vi "Teleop.vi"(10 "Match Info":T1={"Autonomous Elapsed Seconds"=0.0, "TeleOp Elapsed Seconds"=0.0, "Disabled Elapsed Seconds"=0.0, "Visited Autonomous"=FALSE, "Visited TeleOp"=FALSE, "Visited Disabled"=FALSE, "Autonomous Settings"={"Autonomous Style"=enum."Independent", "VI Refnum"=refnum}}, 11 "Call Context":T2) -> ()   [LabVIEW 2015]
doc: "This VI is called for each TeleOp packet received from the DS where the robot is not disabled. It is often used to read from the joysticks and update I/O or to update setpoints for timed control loops. It should complete and return within 20 milliseconds or it may miss DS packets."
uses:
  <vilib>/Rock Robotics/WPI/DriverStation/WPI_DriverStationDerivedRobotMode.ctl
  <vilib>/Rock Robotics/WPI/DriverStation/WPI_DriverStationMatch Info.ctl
  <vilib>/Rock Robotics/WPI/Relay/WPI_RelayValue.ctl
  <vilib>/Rock Robotics/WPI/Utilities/WPI_GetSetVariantRefNum.vi
  <vilib>/Rock Robotics/Network Tables/NT Write Number.vi
  <vilib>/Rock Robotics/Network Tables/NT Write Boolean Array.vi
  <vilib>/Rock Robotics/Network Tables/NT Write Numeric Array.vi
  <vilib>/Rock Robotics/Network Tables/NT Read Number.vi
  Robot Global Data.vi
  <vilib>/Rock Robotics/Network Tables/NT Write Boolean.vi
  <vilib>/Rock Robotics/WPI/RobotDrive/WPI_RobotDriveArcadeDrive_Standard(NoSaturation).vi
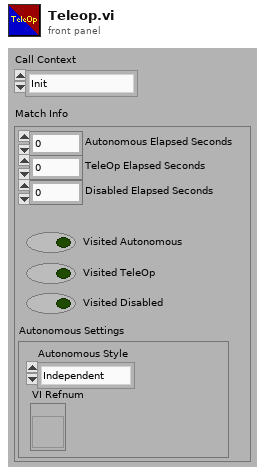
[diagram p1: front panel]
types:
  T1 = typedef "WPI_DriverStationMatch Info.ctl" = cluster{"Autonomous Elapsed Seconds":dbl, "TeleOp Elapsed Seconds":dbl, "Disabled Elapsed Seconds":dbl, "Visited Autonomous":bool, "Visited TeleOp":bool, "Visited Disabled":bool, "Autonomous Settings":cluster{"Autonomous Style":enum16{"Iterative", "Independent"}, "VI Refnum":refnum<vi>}}
  T2 = typedef "WPI_DriverStationDerivedRobotMode.ctl" = enum16{"Init", "Execute", "Stop"}
  T3 = typedef "WPI_RelayValue.ctl" = enum16{"Off", "On", "Forward", "Reverse"}
  T4 = typedef "WPI_JoystickDevRef.ctl" = cluster{"Device":T5}
  T5 = typedef "WPI_JoystickDeviceEnum.ctl" = enum16{"USB 0", "USB 1", "USB 2", "USB 3", "USB 4", "USB 5"}
  T6 = typedef "WPI_ServoDeviceRef.ctl" = cluster{"DeviceStatus":errorcluster, "PWM Channel":T7, "DeadBand":T8}
  T7 = typedef "FPGA_DIOPWMChannel.ctl" = enum8{"PWM 0", "PWM 1", "PWM 2", "PWM 3", "PWM 4", "PWM 5", "PWM 6", "PWM 7", "PWM 8", "PWM 9", "PWM MXP 0", "PWM MXP 1", "PWM MXP 2", "PWM MXP 3", "PWM MXP 4", "PWM MXP 5", "PWM MXP 6", "PWM MXP 7", "PWM MXP 8", "PWM MXP 9", "Invalid"}
  T8 = typedef "WPI_PWMDeadband.ctl" = cluster{"Name":string, "maxPositivePwm":i32, "minPositivePwm":i32, "centerPwm":i32, "maxNegativePwm":i32, "minNegativePwm":i32, "angularRange":u16}
  T9 = typedef "WPI_RobotDriveDevRef.ctl" = cluster{"DevStatus":errorcluster, "Motors[]":T10[], "Square Inputs":bool, "Max Output":dbl}
  T10 = typedef "WPI_MotorControlDeviceRef.ctl" = cluster{"DeviceStatus":errorcluster, "Type":T11, "PWM":cluster{"PWM Channel":T7, "DeadBand":T8}, "CAN":cluster{"Device Number":u8, "Control Mode":T12, "Semaphore":T13, "Max Vout":dbl, "TalonSRX Control Mode":T14}, "Invert":bool}
  T11 = typedef "WPI_MotorControlType.ctl" = enum16{"PWM", "CAN", "CANTalonSRX"}
  T12 = typedef "WPI_CANJaguar_ControlMode.ctl" = enum8{"Percent VBus", "Current", "Speed", "Position", "Voltage"}
  T13 = typedef "Semaphore RefNum" = refnum<k1>
  T14 = typedef "WPI_CANTalonSRX_APIControlMode.ctl" = enum8{"Percent VBus", "Speed", "Position", "Slave", "Unchanged / Invalid", "Voltage Compensation", "Current", "Motion Profile"}
  T15 = typedef "WPI_RelayDevRef.ctl" = cluster{"DevStatus":errorcluster, "Relay Channel":T16, "Relay Direction":T17}
  T16 = typedef "FPGA_DIORelayChannel.ctl" = enum8{"Relay 0", "Relay 1", "Relay 2", "Relay 3", "Invalid"}
  T17 = typedef "WPI_RelayDirection.ctl" = enum16{"Both directions", "Forward only", "Reverse only"}
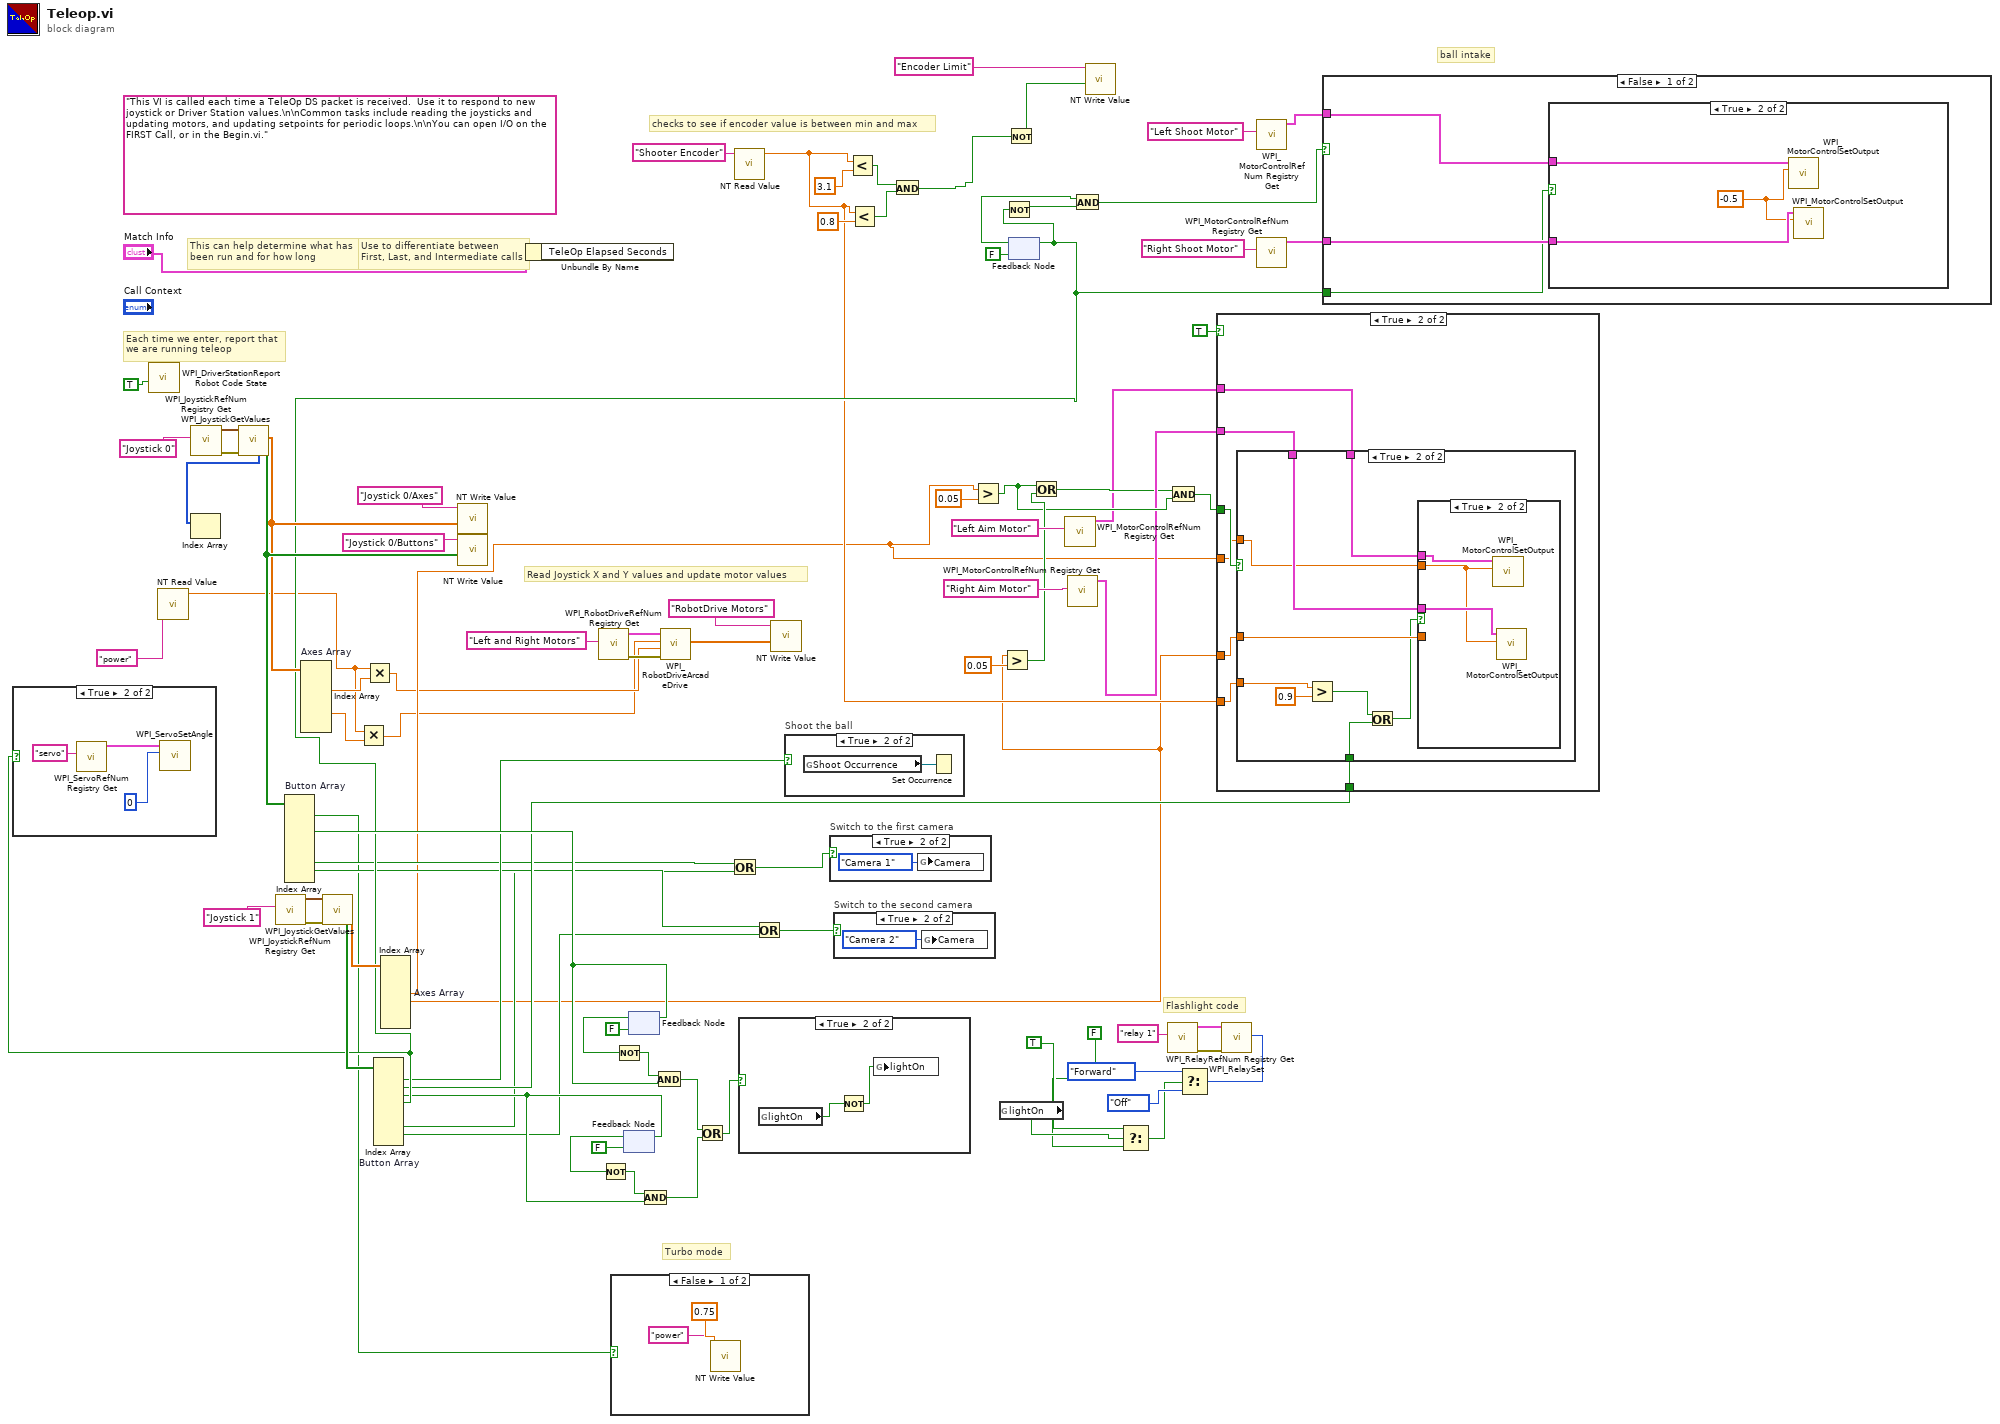
[diagram p0: block diagram]
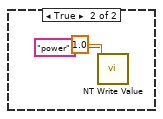
[diagram p2: hidden frame]
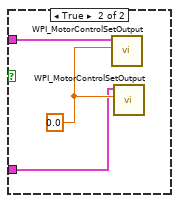
[diagram p5: hidden frame]
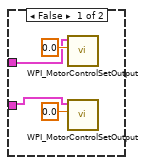
[diagram p7: hidden frame]
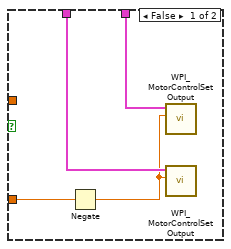
[diagram p8: hidden frame]
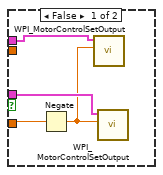
[diagram p9: hidden frame]
diagram:
  (unwired) "This VI is called each time a TeleOp DS packet is received.  Use it to respond to new joystick or Driver Station values.\n\nCommon tasks include reading the joysticks and updating motors, and updating setpoints for periodic loops.\n\nYou can open I/O on the FIRST Call, or in the Begin.vi."
  # "Turbo mode"
  # "ball intake"
  # "Flashlight code"
  # "checks to see if encoder value is between min and max"
  # "Each time we enter, report that\nwe are running teleop"
  # "Use to differentiate between\nFirst, Last, and Intermediate calls"
  # "This can help determine what has\nbeen run and for how long"
  # "Read Joystick X and Y values and update motor values"
  n1 = call <vilib>:"WPI_DriverStationReport Robot Code State.vi"("TeleOp"=TRUE ("Autonomous")) -> ()  [unwired: 10 in, 1 out]
  n2 = call-poly <vilib>:"NT Read Value.vi"("Name"="power") -> ("Numeric"=w3:dbl)  [unwired: 9 in, 1 out]
  n3 = call <vilib>:"WPI_JoystickRefNum Registry Get.vi"("refnum name"="Joystick 0") -> ("error out"=w76:errorcluster, "JoystickDevRef"=w82:T4)  [unwired: 1 in, 8 out]
  n4 = call <vilib>:"WPI_JoystickGetValues.vi"("error in (no error)"=w76, "JoystickDevRef"=w82) -> ("Buttons"=w77:bool[], "Axes"=w74:dbl[], "POVs"=w16:i16[])  [unwired: 5 in, 2 out]
  n5 = Index Array(array=w16) -> ()  [unwired: 1 in, 1 out]
  n6 = call <vilib>:"WPI_JoystickRefNum Registry Get.vi"("refnum name"="Joystick 1") -> ("error out"=w51:errorcluster, "JoystickDevRef"=w53:T4)  [unwired: 1 in, 8 out]
  n7 = Index Array "Button Array"(array=w77) -> (element #1=w9:bool, element #3=w55:bool, element #7=w11:bool, element #8=w14:bool)  [unwired: 9 in, 5 out]
  n8 = Index Array "Axes Array"(array=w74) -> (element #2=w5:dbl, element #5=w2:dbl)  [unwired: 7 in, 5 out]
  n9 = call <vilib>:"WPI_JoystickGetValues.vi"("error in (no error)"=w51, "JoystickDevRef"=w53) -> ("Buttons"=w52:bool[], "Axes"=w50:dbl[])  [unwired: 5 in, 3 out]
  n10 = Multiply(x=w3, y=w2) -> (x*y=w1:dbl)
  n11 = Multiply(x=w3, y=w5) -> (x*y=w4:dbl)
  n12 = Index Array "Button Array"(array=w52) -> (element #1=w26:bool, element #2=w17:bool, element #3=w22:bool, element #4=w27:bool, element #7=w12:bool, element #8=w15:bool)  [unwired: 9 in, 3 out]
  n13 = case shown="True" w27 {
    frame False {
    }
    frame True {
      n14 = call <vilib>:"WPI_ServoRefNum Registry Get.vi"("refnum name"="servo") -> ("ServoDeviceRef"=w89:T6)  [unwired: 9 in, 1 out]
      n15 = call <vilib>:"WPI_ServoSetAngle.vi"("Angle"=0, "ServoDeviceRef"=w89) -> ()  [unwired: 8 in, 2 out]
    }
  }
  n16 = Index Array "Axes Array"(array=w50) -> (element #3=w6:dbl, element #4=w7:dbl)  [unwired: 7 in, 5 out]
  n17 = call-poly <vilib>:"NT Write Value.vi"("Numeric Array"=w74, "Name"="Joystick 0/Axes") -> ()  [unwired: 9 in, 1 out]
  n18 = call-poly <vilib>:"NT Write Value.vi"("Boolean Array"=w77, "Name"="Joystick 0/Buttons") -> ()  [unwired: 9 in, 1 out]
  n19 = Unbundle By Name("Match Info") -> ()  [unwired: 1 out]
  n20 = call <vilib>:"WPI_RobotDriveRefNum Registry Get.vi"("refnum name"="Left and Right Motors") -> ("error out"=w75:errorcluster, "RobotDriveDevRef"=w84:T9)  [unwired: 1 in, 8 out]
  n21 = case shown="False" w9 {
    frame False {
      n22 = call-poly <vilib>:"NT Write Value.vi"("Numeric"=0.75, "Name"="power") -> ()  [unwired: 9 in, 1 out]
    }
    frame True {
      n23 = call-poly <vilib>:"NT Write Value.vi"("Numeric"=1.0, "Name"="power") -> ()  [unwired: 9 in, 1 out]
    }
  }
  n24 = feedback #1(FALSE) -> (w24:bool)
  n25 = Not(x=w24) -> (.not. x?=w23:bool)
  n26 = feedback-in #1(w22) -> ()
  n27 = feedback #2(FALSE) -> (w57:bool)
  n28 = Not(x=w57) -> (.not. x?=w56:bool)
  n29 = feedback-in #2(w55) -> ()
  n30 = And(x=w23, y=w22) -> (x .and. y?=w20:bool)
  n31 = And(x=w56, y=w55) -> (x .and. y?=w21:bool)
  n32 = call-poly <vilib>:"WPI_RobotDriveArcadeDrive.vi"("error in (no error)"=w75, "Y axis value"=w4, "X axis value"=w1, "RobotDriveDevRef"=w84) -> ("Motor Values"=w79:dbl[])  [unwired: 5 in, 2 out]
  n33 = Or(x=w21, y=w20) -> (x .or. y?=w19:bool)
  n34 = Or(x=w11, y=w12) -> (x .or. y?=w10:bool)
  n35 = call-poly <vilib>:"NT Read Value.vi"("Name"="Shooter Encoder" ("refnum name")) -> ("Numeric"=w18:dbl)  [unwired: 9 in, 1 out]
  n36 = case shown="True" w19 {
    frame False {
    }
    frame True {
      n37 = global read "Robot Global Data.vi" "lightOn"() -> (w96:bool)
      n38 = Not(x=w96) -> (.not. x?=w95:bool)
      n39 = global write "Robot Global Data.vi" "lightOn"(w95) -> ()
    }
  }
  n40 = Or(x=w14, y=w15) -> (x .or. y?=w13:bool)
  n41 = call-poly <vilib>:"NT Write Value.vi"("Numeric Array"=w79, "Name"="RobotDrive Motors") -> ()  [unwired: 9 in, 1 out]
  n42 = case "Shoot the ball" shown="True" w26 {
    frame False {
    }
    frame True {
      n43 = global read "Robot Global Data.vi" "Shoot Occurrence"() -> (w97:refnum<k4>)
      n44 = Set Occurrence(w97) -> ()
    }
  }
  n45 = case "Switch to the first camera" shown="True" w10 {
    frame False {
    }
    frame True {
      n46 = global write "Robot Global Data.vi" "Camera"(enum16{"Camera 1", "Camera 2"}."Camera 1" ("Camera")) -> ()
    }
  }
  n47 = case "Switch to the second camera" shown="True" w13 {
    frame False {
    }
    frame True {
      n48 = global write "Robot Global Data.vi" "Camera"(enum16{"Camera 1", "Camera 2"}."Camera 2" ("Camera")) -> ()
    }
  }
  n49 = Less?(x=w18, y=3.1) -> (x < y?=w41:bool)
  n50 = Less?(x=w18, y=0.8) -> (x < y?=w40:bool)
  n51 = And(x=w41, y=w40) -> (x .and. y?=w39:bool)
  n52 = Greater?(x=w6, y=0.05) -> (0:w45:bool)
  n53 = global read "Robot Global Data.vi" "lightOn"() -> (w61:bool)
  n54 = Greater?(x=w7, y=0.05) -> (0:w47:bool)
  n55 = Not(x=w27) -> (.not. x?=w30:bool)
  n56 = Not(x=w39) -> (.not. x?=w69:bool)
  n57 = feedback #3(FALSE) -> (w29:bool)
  n58 = feedback-in #3(w27) -> ()
  n59 = Or(x=w45, y=w47) -> (x .or. y?=w37:bool)
  n60 = call <vilib>:"WPI_MotorControlRefNum Registry Get.vi"("refnum name"="Left Aim Motor") -> ("MotorControlDevRef"=w36:T10)  [unwired: 9 in, 1 out]
  n61 = call <vilib>:"WPI_MotorControlRefNum Registry Get.vi"("refnum name"="Right Aim Motor") -> ("MotorControlDevRef"=w38:T10)  [unwired: 9 in, 1 out]
  n62 = And(x=w29, y=w30) -> (x .and. y?=w28:bool)
  n63 = call-poly <vilib>:"NT Write Value.vi"("Boolean"=w69, "Name"="Encoder Limit") -> ()  [unwired: 9 in, 1 out]
  n64 = Select(t=TRUE, s=w61, f=FALSE) -> (s? t:f=w58:bool)
  n65 = call <vilib>:"WPI_RelayRefNum Registry Get.vi"("refnum name"="relay 1") -> ("error out"=w65:errorcluster, "RelayDevRef"=w66:T15)  [unwired: 9 in]
  n66 = And(x=w37, y=w45) -> (x .and. y?=w44:bool)
  n67 = Select(t=WPI_RelayValue."Forward" ("RelayValue"), s=w58, f=WPI_RelayValue."Off" ("RelayValue")) -> (s? t:f=w62:T3)
  n68 = case shown="True" TRUE {
    tunnel: w38 -> [w101 w109]
    tunnel: w44 -> [_ w110]
    tunnel: w7 -> [_ w108]
    tunnel: w36 -> [w100 w107]
    tunnel: w6 -> [_ w106]
    tunnel: w18 -> [_ w105]
    tunnel: w17 -> [_ w104]
    frame False {
      n69 = call <vilib>:"WPI_MotorControlSetOutput.vi"("Output"=0.0, "MotorControlDevRef"=w100) -> ()  [unwired: 7 in, 3 out]
      n70 = call <vilib>:"WPI_MotorControlSetOutput.vi"("Output"=0.0, "MotorControlDevRef"=w101) -> ()  [unwired: 7 in, 3 out]
    }
    frame True {
      n71 = case shown="True" w110 {
        tunnel: w109 -> [w113 w120]
        tunnel: w108 -> [w112 w119]
        tunnel: w107 -> [w114 w121]
        tunnel: w106 -> [_ w118]
        tunnel: w105 -> [_ w122]
        tunnel: w104 -> [_ w117]
        frame False {
          n72 = Negate(x=w112) -> (-x=w111:dbl)
          n73 = call <vilib>:"WPI_MotorControlSetOutput.vi"("Output"=w111, "MotorControlDevRef"=w114) -> ()  [unwired: 7 in, 3 out]
          n74 = call <vilib>:"WPI_MotorControlSetOutput.vi"("Output"=w111, "MotorControlDevRef"=w113) -> ()  [unwired: 7 in, 3 out]
        }
        frame True {
          n75 = Greater?(x=w122, y=0.9) -> (0:w116:bool)
          n76 = Or(x=w116, y=w117) -> (x .or. y?=w115:bool)
          n77 = case shown="True" w115 {
            tunnel: w121 -> [w127 w130]
            tunnel: w120 -> [w126 w129]
            tunnel: w119 -> [w125 _]
            tunnel: w118 -> [_ w128]
            frame False {
              n78 = Negate(x=w125) -> (-x=w124:dbl)
              n79 = call <vilib>:"WPI_MotorControlSetOutput.vi"("Output"=w124, "MotorControlDevRef"=w127) -> ()  [unwired: 7 in, 3 out]
              n80 = call <vilib>:"WPI_MotorControlSetOutput.vi"("Output"=w124, "MotorControlDevRef"=w126) -> ()  [unwired: 7 in, 3 out]
            }
            frame True {
              n81 = call <vilib>:"WPI_MotorControlSetOutput.vi"("Output"=w128, "MotorControlDevRef"=w130) -> ()  [unwired: 7 in, 3 out]
              n82 = call <vilib>:"WPI_MotorControlSetOutput.vi"("Output"=w128, "MotorControlDevRef"=w129) -> ()  [unwired: 7 in, 3 out]
            }
          }
        }
      }
    }
  }
  n83 = call <vilib>:"WPI_RelaySet.vi"("error in (no error)"=w65, "RelayValue"=w62, "RelayDevRef"=w66) -> ()  [unwired: 7 in, 2 out]
  n84 = call <vilib>:"WPI_MotorControlRefNum Registry Get.vi"("refnum name"="Left Shoot Motor") -> ("MotorControlDevRef"=w33:T10)  [unwired: 9 in, 1 out]
  n85 = call <vilib>:"WPI_MotorControlRefNum Registry Get.vi"("refnum name"="Right Shoot Motor") -> ("MotorControlDevRef"=w32:T10)  [unwired: 9 in, 1 out]
  n86 = case shown="False" w28 {
    tunnel: w33 -> [w133 w138]
    tunnel: w32 -> [w132 w137]
    tunnel: w27 -> [w131 _]
    frame False {
      n87 = case shown="True" w131 {
        tunnel: w133 -> [_ w136]
        tunnel: w132 -> [_ w135]
        frame False {
        }
        frame True {
          w134 = -0.5 ("Output")
          n88 = call <vilib>:"WPI_MotorControlSetOutput.vi"("Output"=w134, "MotorControlDevRef"=w136) -> ()  [unwired: 7 in, 3 out]
          n89 = call <vilib>:"WPI_MotorControlSetOutput.vi"("Output"=w134, "MotorControlDevRef"=w135) -> ()  [unwired: 7 in, 3 out]
        }
      }
    }
    frame True {
      w139 = 0.0 ("Output")
      n90 = call <vilib>:"WPI_MotorControlSetOutput.vi"("Output"=w139, "MotorControlDevRef"=w138) -> ()  [unwired: 7 in, 3 out]
      n91 = call <vilib>:"WPI_MotorControlSetOutput.vi"("Output"=w139, "MotorControlDevRef"=w137) -> ()  [unwired: 7 in, 3 out]
    }
  }
